vi "WWVB to time.vi"(11 "WWVB":u64 format="%.0x") -> ()   [LabVIEW 2019]
panel:
  out "output 1":timestamp
  # "10C2708D0210823"
  # "1182708D0210825"
  # "2202708D0210823"
  # "2842708D0210823"
  # "880308D2210823"
  # "1000308D2210823"
  # "1040308D2210823"
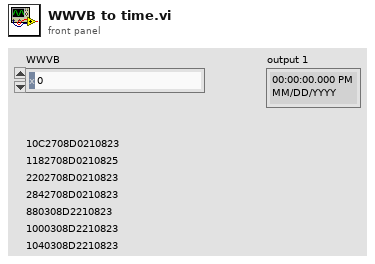
[diagram p1: front panel]
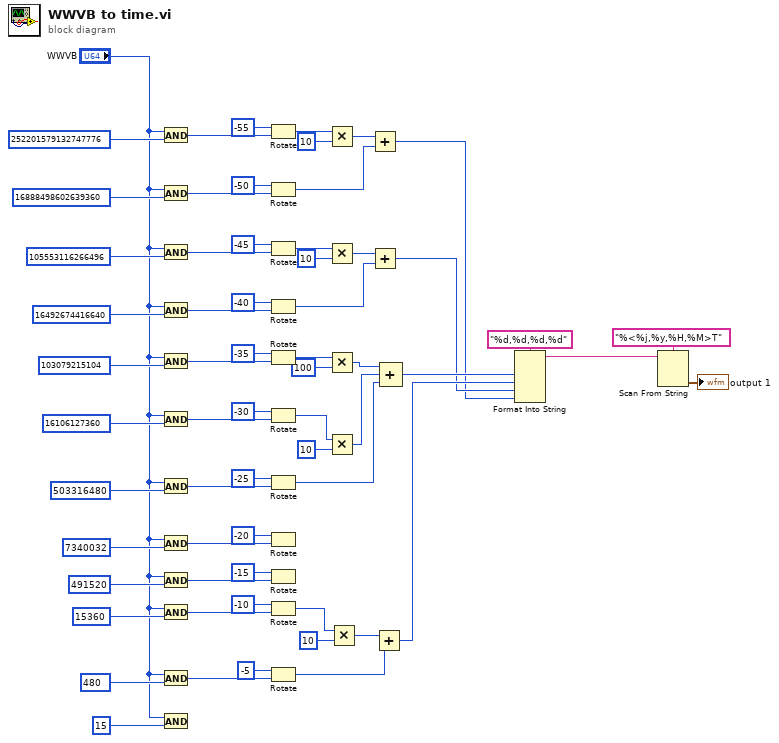
[diagram p0: block diagram]
diagram:
  n1 = And(x="WWVB", y=u64 252201579132747776) -> (x .and. y?=w57:u64)
  n2 = And(x="WWVB", y=u64 16888498602639360) -> (x .and. y?=w60:u64)
  n3 = And(x="WWVB", y=u64 105553116266496) -> (x .and. y?=w50:u64)
  n4 = And(x="WWVB", y=u64 16492674416640) -> (x .and. y?=w47:u64)
  n5 = And(x="WWVB", y=u64 103079215104) -> (x .and. y?=w37:u64)
  n6 = And(x="WWVB", y=u64 16106127360) -> (x .and. y?=w40:u64)
  n7 = And(x="WWVB", y=u64 503316480) -> (x .and. y?=w30:u64)
  n8 = And(x="WWVB", y=u64 7340032) -> (x .and. y?=w26:u64)
  n9 = And(x="WWVB", y=u64 491520) -> (x .and. y?=w21:u64)
  n10 = And(x="WWVB", y=u64 15360) -> (x .and. y?=w20:u64)
  n11 = And(x="WWVB", y=u64 480) -> (x .and. y?=w14:u64)
  n12 = And(x="WWVB", y=u64 15) -> ()  [unwired: 1 out]
  n13 = Rotate(1:w57, 2:i16 -55 ("y")) -> (0:w56:u64)
  n14 = Rotate(1:w60, 2:i16 -50 ("y")) -> (0:w53:u64)
  n15 = Rotate(1:w50, 2:i16 -45 ("y")) -> (0:w51:u64)
  n16 = Rotate(1:w47, 2:i16 -40 ("y")) -> (0:w43:u64)
  n17 = Rotate(1:w37, 2:i16 -35 ("y")) -> (0:w36:u64)
  n18 = Rotate(1:w40, 2:i16 -30 ("y")) -> (0:w33:u64)
  n19 = Rotate(1:w30, 2:i16 -25 ("y")) -> (0:w27:u64)
  n20 = Rotate(1:w26, 2:i16 -20 ("y")) -> ()  [unwired: 1 out]
  n21 = Rotate(1:w21, 2:i16 -15 ("y")) -> ()  [unwired: 1 out]
  n22 = Rotate(1:w20, 2:i16 -10 ("y")) -> (0:w16:u64)
  n23 = Rotate(1:w14, 2:i16 -5 ("y")) -> (0:w12:u64)
  n24 = Multiply(x=w56, y=u64 10) -> (x*y=w54:u64)
  n25 = Multiply(x=w51, y=u64 10) -> (x*y=w44:u64)
  n26 = Multiply(x=w36, y=u64 100) -> (x*y=w29:u64)
  n27 = Multiply(x=w33, y=u64 10) -> (x*y=w28:u64)
  n28 = Multiply(x=w16, y=u64 10) -> (x*y=w13:u64)
  n29 = Add(x=w54, y=w53) -> (x+y=w1:u64)
  n30 = Add(x=w44, y=w43) -> (x+y=w2:u64)
  n31 = Add(x=w13, y=w12) -> (x+y=w3:u64)
  n32 = Compound Arithmetic op=ADD(w29, w28, w27) -> (w4:u64)
  n33 = Format Into String(format string="%d,%d,%d,%d", w4, w3, w2, w1) -> (resulting string=w5:string)  [unwired: 2 in, 1 out]
  n34 = Scan From String(format string="%<%j,%y,%H,%M>T", input string=w5) -> (output 1=→"output 1":timestamp)  [unwired: 3 in, 3 out]
